vi "Populate Tree with Message Array.vi"(8 "error in (no error)":errorcluster, 10 "Message Array":refnum<class "Message.lvclass">[](array[class]), 11 "Tree in":refnum<vi>) -> (0 "error out":errorcluster, 3 "Tree out":refnum<vi>)   [LabVIEW 2020, in "Sequencer.lvlib"]
doc: "Populate a Tree Control with message base names. The tree is indented when a child of the Batch Msg is encountered. Any previous element will be removed from the tree before the Message Array is added."
uses:
  Sequencer.lvlib
  PPL/HDH.Actor Framework.Core.Actor.lvlibp/1abvi3w/vi.lib/ActorFramework/Message/Message.lvclass
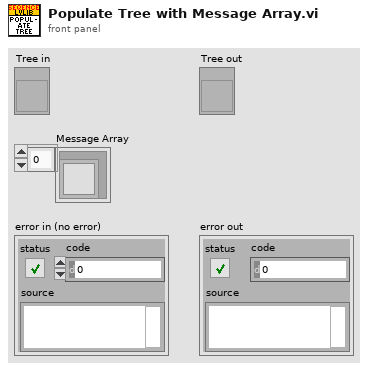
[diagram p1: front panel]
types:
  T1 = cluster{"Left Cell String":string, "Child Text":string[], "Child Tag":string, "Item Indent":i32, "Child Only?":bool, "Glyph Index":i32}
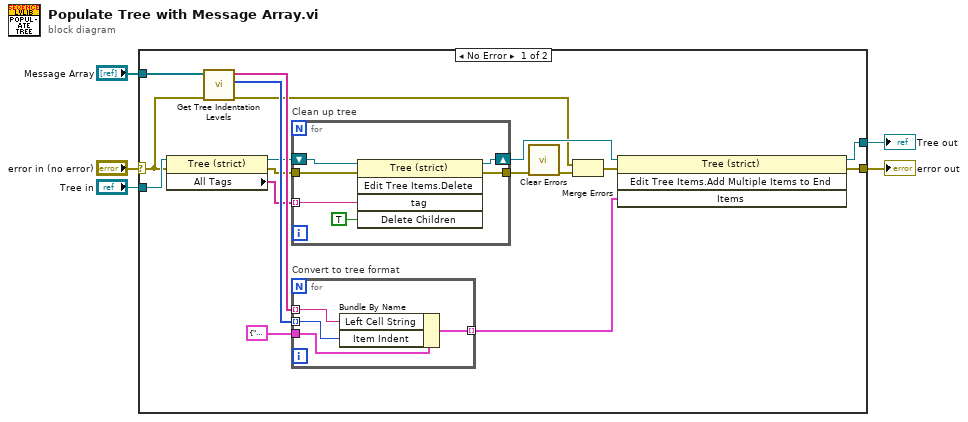
[diagram p0: block diagram]
diagram:
  n1 = case shown="No Error" "error in (no error)" {
    selector: "error in (no error)" -> [w10 w33]
    tunnel: "Message Array" -> [w22 _]
    tunnel: "Tree in" -> [w14 w34]
    tunnel: [w11 w33] -> w3
    tunnel: [w9 w34] -> w5
    frame No Error {
      n2 = property on="Property Node" class="Tree (strict)"(reference=w14, error in=w10) -> (reference out=w13:refnum<vi>, error out=w8:errorcluster, "All Tags"=w17:string[])
      n3 = call "Get Tree Indentation Levels.vi"("error in (no error)"=w10, "Message Array"=w22) -> ("error out"=w6:errorcluster, "Tree indentation level Array"=w19:i32[], "Class Base Name Array"=w20:string[])  [unwired: 7 in]
      n4 = for "Clean up tree" {
        tunnel: w17 -> [w28] mode=indexing
        tunnel: [w26] -> w16
        shift-right: [w24] -> w12
        shift-left: w13 -> [w25]
        tunnel: w8 -> [w23]
        n5 = invoke on="Invoke Node" class="Tree (strict)" method="Edit Tree Items.Delete"(reference=w25, error in=w23, "tag"=w28, "Delete Children"=TRUE ("Delete Children?")) -> (reference out=w24:refnum<vi>, error out=w26:errorcluster)  [unwired: 1 in, 3 out]
      }
      n6 = for "Convert to tree format" {
        tunnel: T1 {"Left Cell String"="", "Child Text"=[], "Child Tag"="", "Item Indent"=0, "Child Only?"=FALSE, "Glyph Index"=0} ("Item") -> [w32]
        tunnel: w20 -> [w31] mode=indexing
        tunnel: w19 -> [w30] mode=indexing
        tunnel: [w29] -> w18 mode=indexing
        n7 = Bundle By Name(cluster=w32, "Left Cell String"=w31, "Item Indent"=w30) -> (w29:T1)
      }
      n8 = call <vilib>:"Clear Errors.vi"("error in (no error)"=w16) -> ("error out"=w15:errorcluster)  [unwired: 5 in, 1 out]
      n9 = Merge Errors(w6, w15) -> (w7:errorcluster)
      n10 = invoke on="Invoke Node" class="Tree (strict)" method="Edit Tree Items.Add Multiple Items to End"(reference=w12, error in=w7, "Items"=w18) -> (reference out=w9:refnum<vi>, error out=w11:errorcluster)  [unwired: 1 in, 2 out]
    }
    frame Error {
    }
  }
  "Tree out" <- w5
  "error out" <- w3
